vi "DOE Washer HCC AGILENT Scale.vi"(0 "Headers":string[](array[string]), 5 "Agilent Data Input":dbl[](array[numeric]), 7 "Voltage Scale":dbl=30.0 format="%#_13g", 9 "Current Scale":dbl=2.0 format="%#_13g", 11 "Error In":errorcluster, 12 "Pressure Scale":dbl=30.0 format="%#_13g") -> (4 "Scaled Output Data":string[](array[string]), 15 "Error Out":errorcluster)   [LabVIEW 2019]
uses:
  <vilib>/Utility/error.llb/whitespace.ctl
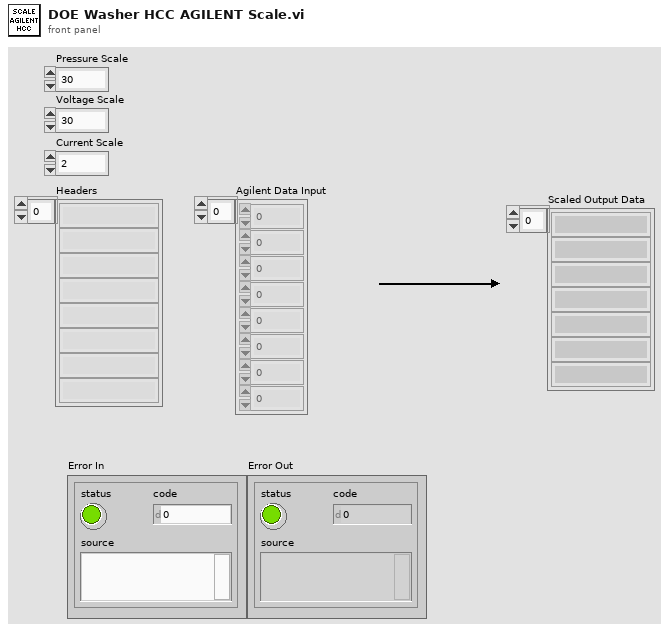
[diagram p1: front panel]
types:
  T1 = typedef "whitespace.ctl" = u16
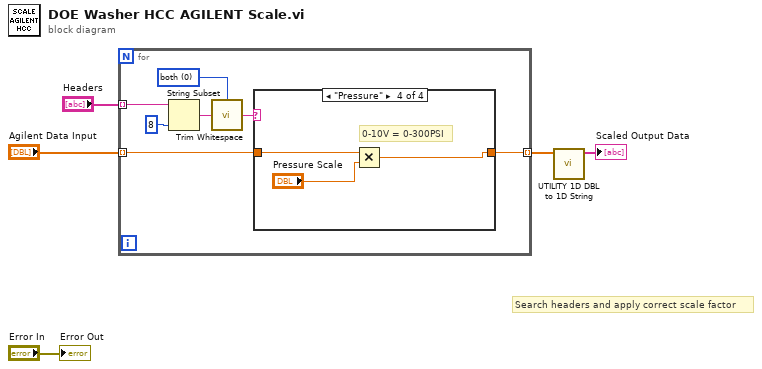
[diagram p0: block diagram]
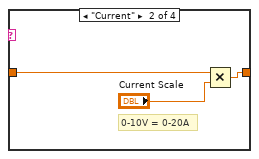
[diagram p3: hidden frame]
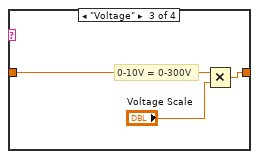
[diagram p4: hidden frame]
diagram:
  # "Search headers and apply correct scale factor"
  n1 = for {
    tunnel: "Agilent Data Input" -> [w7] mode=indexing
    tunnel: "Headers" -> [w8] mode=indexing
    tunnel: [w6] -> w3 mode=indexing
    w12 = T1 0 items=["both", "start of string", "end of string"] ("location (both)")
    n2 = String Subset(string=w8, length (rest)=8 ("length (rest)")) -> (substring=w11:string)  [unwired: 1 in]
    n3 = call <vilib>:"Trim Whitespace.vi"("string"=w11, "location (both)"=w12) -> ("trimmed string"=w9:string)
    n4 = case shown="\"Pressure\"" w9 {
      tunnel: w7 -> [w13 w15 w19 w20]
      tunnel: [w13 w14 w18 w21] -> w6
      frame "False", Default {
      }
      frame "Current" {
        # "0-10V = 0-20A"
        n5 = Multiply(x=w15, y="Current Scale") -> (x*y=w14:dbl)
      }
      frame "Voltage" {
        # "0-10V = 0-300V"
        n6 = Multiply(x=w19, y="Voltage Scale") -> (x*y=w18:dbl)
      }
      frame "Pressure" {
        # "0-10V = 0-300PSI"
        n7 = Multiply(x=w20, y="Pressure Scale") -> (x*y=w21:dbl)
      }
    }
  }
  n8 = call "UTILITY 1D DBL to 1D String.vi"("1D DBL"=w3) -> ("1D String"=→"Scaled Output Data":string[])  [unwired: 10 in]
  "Error Out" <- "Error In"
